vi "pl1000Open.vi"(8 "error in (no error)":errorcluster) -> (0 "error out":errorcluster, 1 "UnitInfo":T1, 2 "maxValue":u16, 3 "pl1000 handle out":i16)   [LabVIEW 2010]
uses:
  pl1000.dll
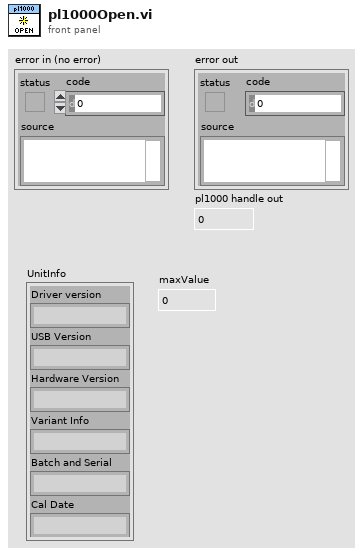
[diagram p1: front panel]
types:
  T1 = cluster{"Driver version":string, "USB Version":string, "Hardware Version":string, "Variant Info":string, "Batch and Serial":string, "Cal Date":string, "[6]":string, "[7]":string, "[8]":string}
  T2 = cluster{"status":bool, "code":u32, "source":string}
  T3 = cluster{"status":bool, "code":bool, "source":bool}
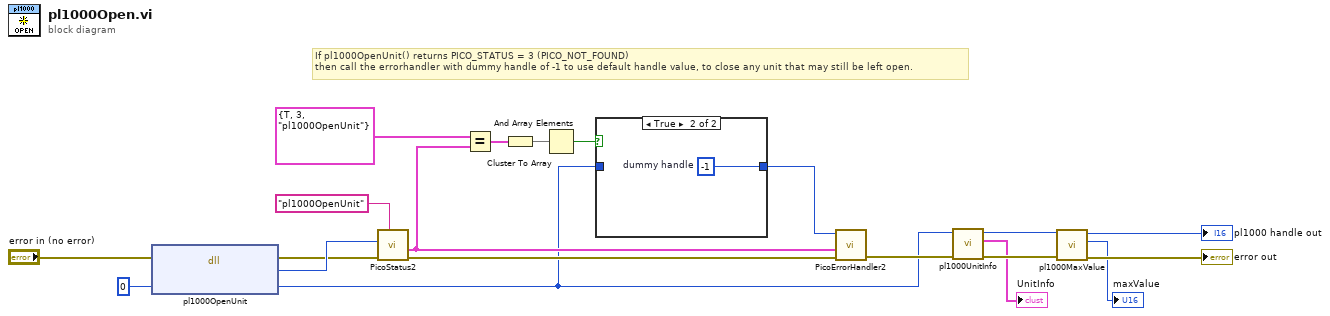
[diagram p0: block diagram]
diagram:
  # "If pl1000OpenUnit() returns PICO_STATUS = 3 (PICO_NOT_FOUND)\nthen call the errorhandler with dummy handle of -1 to use default handle value, to close any unit that may still be left open."
  n1 = dll-call lib="pl1000.dll" fn="pl1000OpenUnit"(error in="error in (no error)", "handle"=i16 0) -> (error out=w17:errorcluster, "status"=w18:u32, "handle"=w2:i16)  [unwired: 2 in, 1 out]
  n2 = call "PicoStatus2.vi"("PICO source"="pl1000OpenUnit", "Error in"=w17, "PICO STATUS"=w18) -> ("error out"=w13:errorcluster, "PICO_STATUS out"=w12:T2)  [unwired: 5 in]
  n3 = Equal?(x=T2 {"status"=TRUE, "code"=3, "source"="pl1000OpenUnit"} ("PICO_STATUS out"), y=w12) -> (x = y?=w15:T3)
  n4 = Cluster To Array(cluster=w15) -> (array=w14:bool[])
  n5 = And Array Elements(Boolean array=w14) -> (logical AND=w11:bool)
  n6 = case shown="True" w11 {
    tunnel: w2 -> [w21 _]
    tunnel: [w21 w22] -> w10
    frame False {
    }
    frame True {
      w22 = i16 -1  # dummy handle
    }
  }
  n7 = call "PicoErrorHandler2.vi"("error in (no error)"=w13, "PICO_STATUS in"=w12, "handle In"=w10) -> ("error out"=w4:errorcluster)  [unwired: 8 in]
  n8 = call "pl1000UnitInfo.vi"("error in (no error)"=w4, "pl1000 handle"=w2) -> ("error out"=w5:errorcluster, "UnitInfo"=→"UnitInfo":T1, "pl1000 handle out"=w3:i16)  [unwired: 7 in]
  n9 = call "pl1000MaxValue.vi"("error in (no error)"=w5, "pl1000 handle"=w3) -> ("error out"=→"error out":errorcluster, "maxValue"=→"maxValue":u16, "pl1000 handle out"=→"pl1000 handle out":i16)  [unwired: 7 in]
